vi "WriteString.vi"(8 "error in (no error)":errorcluster, 9 "Standard":string, 10 "BW":string, 11 "refnum out":refnum<file>) -> (0 "error out":errorcluster, 3 "refnum out 2":refnum<file>)   [LabVIEW 2012]
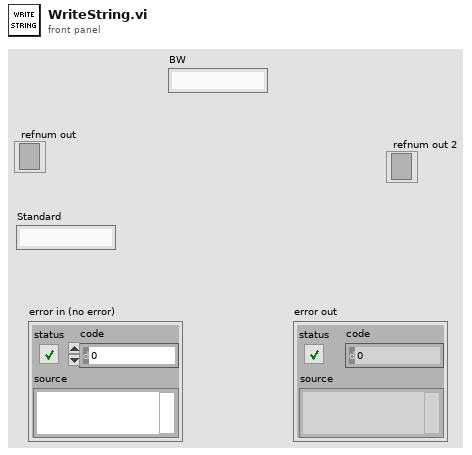
[diagram p1: front panel]
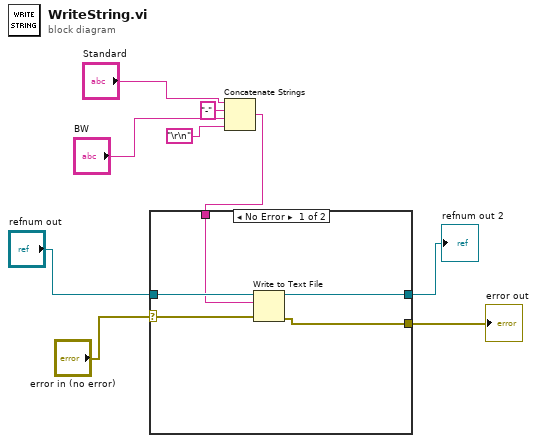
[diagram p0: block diagram]
diagram:
  n1 = Concatenate Strings("Standard", "-" ("string"), "BW", "\r\n") -> (w4:string)
  n2 = case shown="No Error" "error in (no error)" {
    selector: "error in (no error)" -> [w13 w15]
    tunnel: [w12 w15] -> w8
    tunnel: "refnum out" -> [w14 _]
    tunnel: w4 -> [w11 _]
    tunnel: [w10 _] -> w6
    frame No Error {
      n3 = Write to Text File(file (use dialog)=w14, text=w11, error in=w13) -> (refnum out=w10:refnum<file>, error out=w12:errorcluster)  [unwired: 1 in, 1 out]
    }
    frame Error {
    }
  }
  "error out" <- w8
  "refnum out 2" <- w6
